vi "Control_Score.vi"(8 "Player":T1) -> ()   [LabVIEW 2018]
uses:
  TypDefs/Player_Enum.ctl
  <vilib>/rvi/Emulation/niFpgaGetClockAttributes.vi
  <vilib>/rvi/Emulation/niFpgaSctlEmulationGetInTimedLoop.vi
  <vilib>/rvi/Emulation/niFpgaEmulationReportErrorSimple.vi
  Global_GameOver.vi
  Game/Global_ScorePlayer1.vi
  Game/Global_ScorePlayer2.vi
  <vilib>/rvi/Memory/Memory_Emulation/nirvimemoryFastEmulation.vi
  <vilib>/rvi/Memory/Memory_Emulation/nirvimemoryEmulation.vi
  <vilib>/rvi/Emulation/niFpgaEmulationIsFPGAContextNoSignature.vi
  <vilib>/rvi/DataTransferAndStorage/Container/Common/niFpgaContainerGetUniqueNameForEmu.vi
  <vilib>/rvi/Emulation/niFpgaProcessEmulError.vi
  <vilib>/rvi/errors/nirviReportUnexpectedCaseInternalError (U32).vi
  <vilib>/rvi/Emulation/niFpgaCriticalErrorInLSC.vi
  <vilib>/rvi/DataTransferAndStorage/Container/XNode/niFpgaContainer.xnode
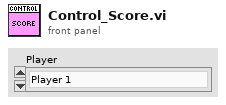
[diagram p1: front panel]
types:
  T1 = typedef "Player_Enum.ctl" = enum16{"Player 1", "Player 2"}
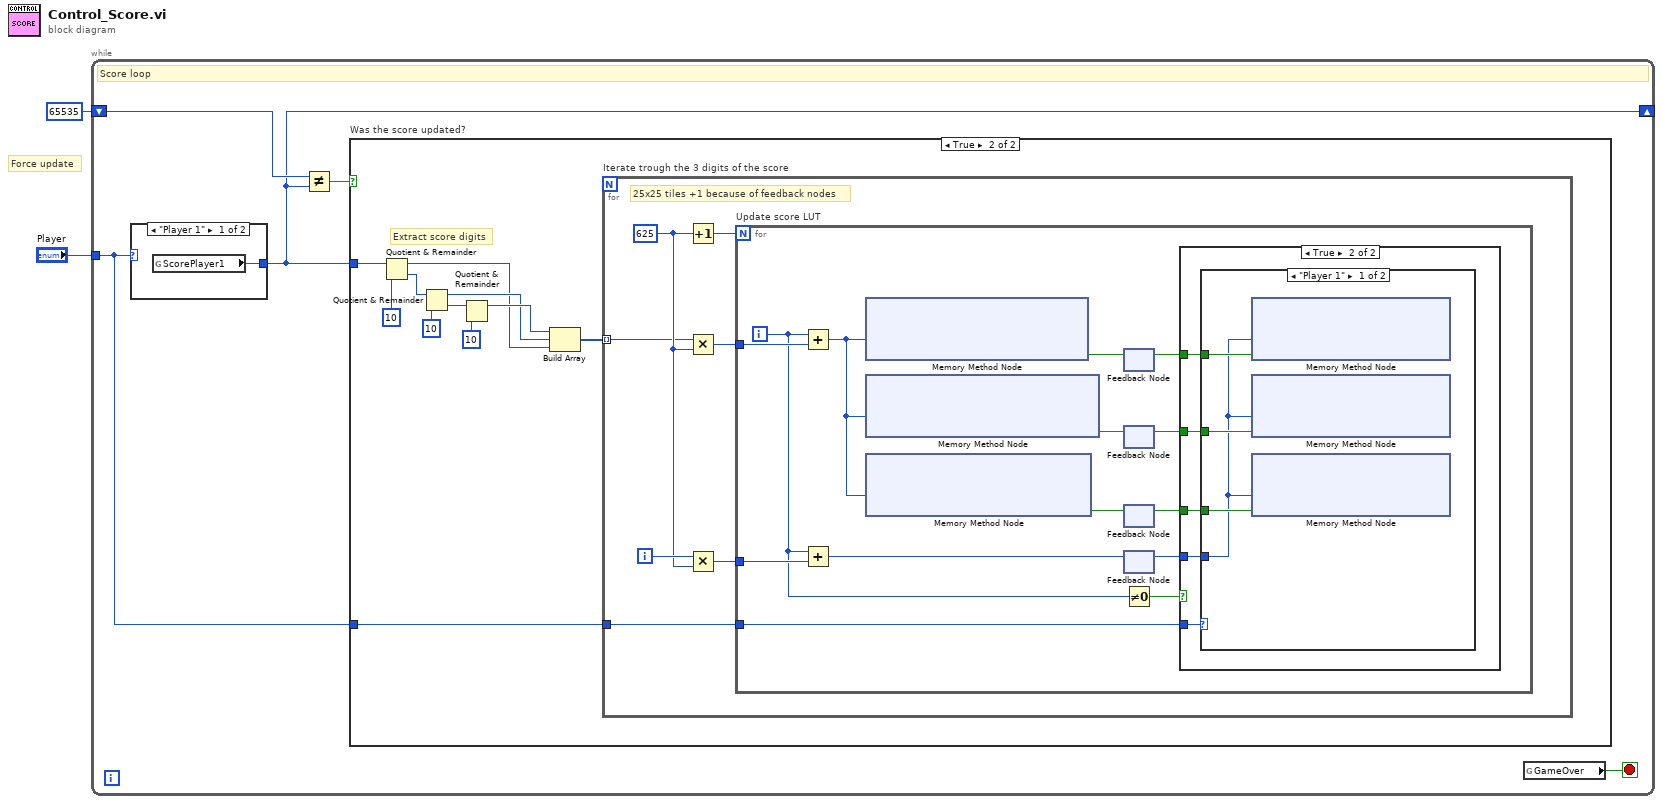
[diagram p0: block diagram]
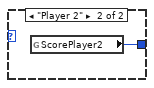
[diagram p2: hidden frame]
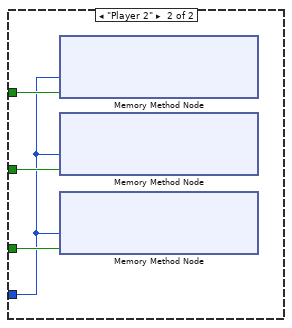
[diagram p5: hidden frame]
diagram:
  # "Force update"
  n1 = while {
    shift-right: [w4] -> _
    shift-left: u16 65535 ("ScorePlayer1") -> [w6]
    tunnel: "Player" -> [w3]
    stop <- w7 stop-if-true
    # "Score loop"
    n2 = case shown="\"Player 1\"" w3 {
      tunnel: [w8 w9] -> w4
      frame "Player 1" {
        n3 = global read "Global_ScorePlayer1.vi" "ScorePlayer1"() -> (w8:u16)
      }
      frame "Player 2" {
        n4 = global read "Global_ScorePlayer2.vi" "ScorePlayer2"() -> (w9:u16)
      }
    }
    n5 = Not Equal?(x=w6, y=w4) -> (x != y?=w5:bool)
    n6 = case "Was the score updated?" shown="True" w5 {
      tunnel: w4 -> [_ w17]
      tunnel: w3 -> [_ w10]
      frame False {
      }
      frame True {
        # "Extract score digits"
        n7 = Quotient & Remainder(x=w17, y=u16 10) -> (x-y*floor(x/y)=w11:u16, floor(x/y)=w19:u16)
        n8 = Quotient & Remainder(x=w19, y=u16 10) -> (x-y*floor(x/y)=w12:u16, floor(x/y)=w18:u16)
        n9 = Quotient & Remainder(x=w18, y=u16 10) -> (x-y*floor(x/y)=w13:u16)  [unwired: 1 out]
        n10 = Build Array(w13, w12, w11) -> (w20:u16[])
        n11 = for "Iterate trough the 3 digits of the score" {
          tunnel: w20 -> [w23] mode=indexing
          tunnel: w10 -> [w21]
          i -> [w27]
          w25 = 625
          # "25x25 tiles +1 because of feedback nodes"
          n12 = Increment(x=w25) -> (x+1=w22:i32)
          n13 = Multiply(x=w23, y=w25) -> (x*y=w24:i32)
          n14 = Multiply(x=w27, y=w25) -> (x*y=w26:i32)
          n15 = for "Update score LUT" {
            N: w22 -> [_]
            tunnel: w26 -> [w35]
            tunnel: w24 -> [w33]
            tunnel: w21 -> [w28]
            i -> [w30]
            n16 = Add(x=w30, y=w33) -> (x+y=w32:i32)
            n17 = Add(x=w30, y=w35) -> (x+y=w34:i32)
            n18 = xnode ("Memory Method Node")("Address A"=w32) -> ("Data A"=w41:bool)  [unwired: 1 in, 1 out]
            n19 = xnode ("Memory Method Node")("Address A"=w32) -> ("Data A"=w40:bool)  [unwired: 1 in, 1 out]
            n20 = xnode ("Memory Method Node")("Address A"=w32) -> ("Data A"=w39:bool)  [unwired: 1 in, 1 out]
            n21 = feedback #1() -> (w38:bool)  [unwired: 1 in]
            n22 = feedback-in #1(w41) -> ()
            n23 = feedback #2() -> (w37:bool)  [unwired: 1 in]
            n24 = feedback-in #2(w40) -> ()
            n25 = feedback #3() -> (w36:bool)  [unwired: 1 in]
            n26 = feedback-in #3(w39) -> ()
            n27 = feedback #4() -> (w31:i32)  [unwired: 1 in]
            n28 = feedback-in #4(w34) -> ()
            n29 = Not Equal To 0?(x=w30) -> (x != 0?=w29:bool)
            n30 = case shown="True" w29 {
              tunnel: w38 -> [_ w46]
              tunnel: w37 -> [_ w45]
              tunnel: w36 -> [_ w44]
              tunnel: w31 -> [_ w43]
              tunnel: w28 -> [_ w42]
              frame False {
              }
              frame True {
                n31 = case shown="\"Player 1\"" w42 {
                  tunnel: w46 -> [w50 w54]
                  tunnel: w45 -> [w49 w53]
                  tunnel: w44 -> [w48 w52]
                  tunnel: w43 -> [w47 w51]
                  frame "Player 1" {
                    n32 = xnode ("Memory Method Node")("Address"=w47, "Data"=w50) -> ()  [unwired: 1 in, 1 out]
                    n33 = xnode ("Memory Method Node")("Address"=w47, "Data"=w49) -> ()  [unwired: 1 in, 1 out]
                    n34 = xnode ("Memory Method Node")("Address"=w47, "Data"=w48) -> ()  [unwired: 1 in, 1 out]
                  }
                  frame "Player 2" {
                    n35 = xnode ("Memory Method Node")("Address"=w51, "Data"=w54) -> ()  [unwired: 1 in, 1 out]
                    n36 = xnode ("Memory Method Node")("Address"=w51, "Data"=w53) -> ()  [unwired: 1 in, 1 out]
                    n37 = xnode ("Memory Method Node")("Address"=w51, "Data"=w52) -> ()  [unwired: 1 in, 1 out]
                  }
                }
              }
            }
          }
        }
      }
    }
    n38 = global read "Global_GameOver.vi" "GameOver"() -> (w7:bool)
  }
